vi "Force Unreserve Resource.vi"(8 "error in (no error)":errorcluster, 10 "Name in bitfile":string, 11 "Item Ref in":T1 format="%.0x") -> (0 "error out":errorcluster, 3 "Item Ref out":T1 format="%.0x")   [LabVIEW 2016, in "FPGA RM System Definition API.lvlib"]
uses:
  FPGA RM System Definition API.lvlib
  <vilib>/NI Veristand/Custom Device API/Custom Device Item Ref.ctl
  <vilib>/NI VeriStand/Custom Device API/Custom Device API.lvlib
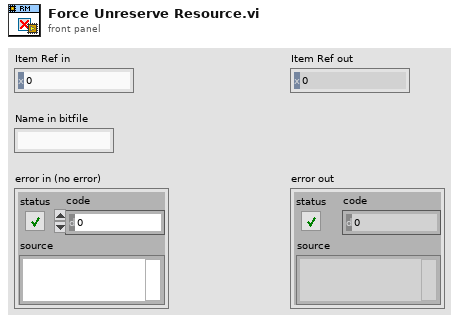
[diagram p1: front panel]
types:
  T1 = typedef "Custom Device API.lvlib/Custom Device Item Ref.ctl" = u64
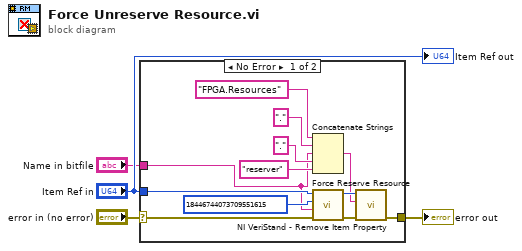
[diagram p0: block diagram]
diagram:
  n1 = case shown="No Error" "error in (no error)" {
    selector: "error in (no error)" -> [w14 w17]
    tunnel: [w12 w17] -> w3
    tunnel: "Item Ref in" -> [w16 _]
    tunnel: "Name in bitfile" -> [w7 _]
    frame No Error {
      n2 = Concatenate Strings("FPGA.Resources" ("string"), "." ("string"), w7, "." ("string"), "reserver" ("string")) -> (w6:string)
      n3 = call "Force Reserve Resource.vi"("error in (no error)"=w14, "Name in bitfile"=w7, "Client Node Ref"=T1 18446744073709551615, "Item Ref in"=w16) -> ("error out"=w13:errorcluster, "Item Ref out"=w11:T1)  [unwired: 6 in]
      n4 = call <vilib>:"NI VeriStand - Remove Item Property.vi"("error in (no error)"=w13, "Property Name"=w6, "Item Ref in"=w11) -> ("error out"=w12:errorcluster)  [unwired: 6 in, 2 out]
    }
    frame Error {
    }
  }
  "error out" <- w3
  "Item Ref out" <- "Item Ref in"
